vi "3b_lit_TXT.vi"(4 "err in":errorcluster, 6 "src":T1, 7 "tdms in":refnum<k34>) -> (0 "err out":errorcluster, 1 "do_txt":T5, 2 "src":T1, 3 "tdms out":refnum<k34>)   [LabVIEW 2010, in "lv_04.lvlib"]
uses:
  lv_04.lvlib
  commandes/cSTA_varid.ctl
  commandes/c_TDMS_ch_variable.ctl
  commandes/c_TDMS_ch_donnees.ctl
  commandes/c0-var-n.ctl
  commandes/c02-do-txt.ctl
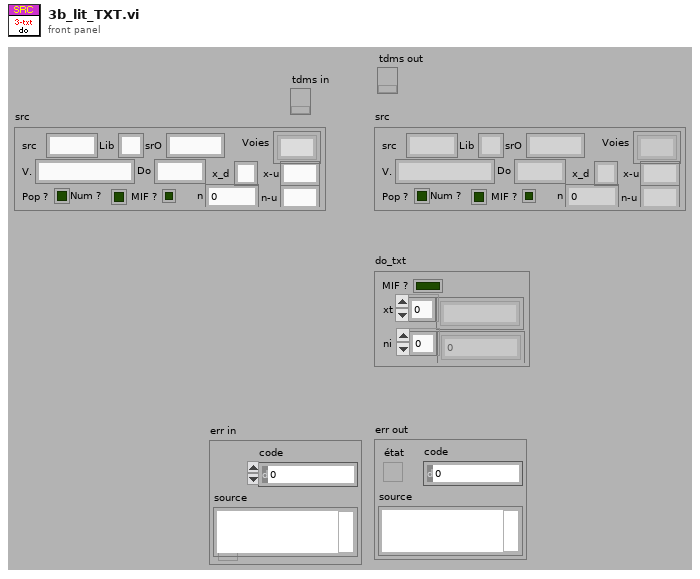
[diagram p1: front panel]
types:
  T1 = typedef "lv_04.lvlib/cSTA_varid.ctl" = cluster{"src":string, "Lib":string, "srO":string, "V.":T2, "Voies":string[], "Do":T3, "n":T4, "Num ?":bool, "Pop ?":bool, "x_d":string, "x-u":string, "n-u":string, "MIF ?":bool}
  T2 = typedef "lv_04.lvlib/c_TDMS_ch_variable.ctl" = string
  T3 = typedef "lv_04.lvlib/c_TDMS_ch_donnees.ctl" = string
  T4 = typedef "lv_04.lvlib/c0-var-n.ctl" = i32
  T5 = typedef "lv_04.lvlib/c02-do-txt.ctl" = cluster{"xt":string[], "ni":dbl[], "MIF ?":bool}
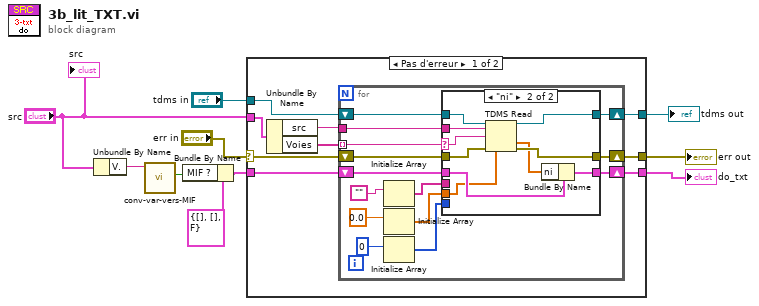
[diagram p0: block diagram]
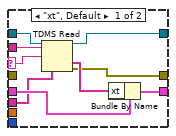
[diagram p2: hidden frame]
diagram:
  n1 = Unbundle By Name("src") -> ("V."=w4:T2)
  n2 = call "conv-var-vers-MIF.vi"("Variable"=w4) -> ("MIF ?"=w3:bool)  [unwired: 4 in, 2 out]
  n3 = Bundle By Name(cluster=T5 {"xt"=[], "ni"=[], "MIF ?"=FALSE} ("X_txt 2"), "MIF ?"=w3) -> (w1:T5)
  n4 = case shown="Pas d'erreur" "err in" {
    selector: "err in" -> [w18 w53]
    tunnel: "tdms in" -> [w19 w55]
    tunnel: [w17 w55] -> w8
    tunnel: "src" -> [w16 _]
    tunnel: [w15 w54] -> w6
    tunnel: w1 -> [w14 w54]
    tunnel: [w11 w53] -> w7
    frame No Error {
      n5 = Unbundle By Name(w16) -> ("src"=w12:string, "Voies"=w13:string[])
      n6 = for {
        tunnel: w13 -> [w33] mode=indexing
        tunnel: w12 -> [w29]
        shift-right: [w27] -> w11
        shift-left: w18 -> [w26]
        shift-right: [w20] -> w15
        shift-left: w14 -> [w21]
        shift-right: [w25] -> w17
        shift-left: w19 -> [w28]
        n7 = Initialize Array("") -> (w31:string[])  [unwired: 1 in]
        n8 = Initialize Array(0.0) -> (w30:dbl[])  [unwired: 1 in]
        n9 = Initialize Array(0) -> (w22:i32[])  [unwired: 1 in]
        n10 = case shown="\"ni\"" w33 {
          selector: w33 -> [w36 w50]
          tunnel: w31 -> [w37 _]
          tunnel: w30 -> [_ w43]
          tunnel: w29 -> [w42 w51]
          tunnel: w28 -> [w35 w52]
          tunnel: [w38 w48] -> w27
          tunnel: w26 -> [_ w49]
          tunnel: [w34 w45] -> w25
          tunnel: w22 -> [_ _]
          tunnel: w21 -> [w41 w47]
          tunnel: [w40 w44] -> w20
          frame "xt", Default {
            n11 = TDMS Read(0:w35, 5:w42, 7:w36, 12:w37) -> (4:w34:refnum<k34>, 10:w39:string[], 15:w38:errorcluster)  [unwired: 3 in, 3 out]
            n12 = Bundle By Name(cluster=w41, "xt"=w39) -> (w40:T5)
          }
          frame "ni" {
            n13 = TDMS Read(0:w52, 5:w51, 7:w50, 11:w49, 12:w43) -> (4:w45:refnum<k34>, 10:w46:dbl[], 15:w48:errorcluster)  [unwired: 2 in, 3 out]
            n14 = Bundle By Name(cluster=w47, "ni"=w46) -> (w44:T5)
          }
        }
      }
    }
    frame Error {
    }
  }
  "err out" <- w7
  "tdms out" <- w8
  "do_txt" <- w6
  "src" <- "src"
